vi "Write ACQ Data.vi"(8 "error in (no error)":errorcluster, 10 "ACQ Data":T1, 11 "DriverMasterAsync in":refnum<class "DriverMasterAsync.lvclass">) -> (0 "error out":errorcluster, 3 "DriverMasterAsync out":refnum<class "DriverMasterAsync.lvclass">)   [LabVIEW 2014, in "DriverMasterAsync.lvlib" / "DriverMasterAsync.lvclass"]
uses:
  DriverMasterAsync.lvclass
  APIs/Data Queue/Async Acquisition Data Cluster.ctl
  DriverMasterAsync.lvclass/DriverMasterAsync.ctl
  APIs/Data Queue/WINFAS 2 Data Queue.lvlib
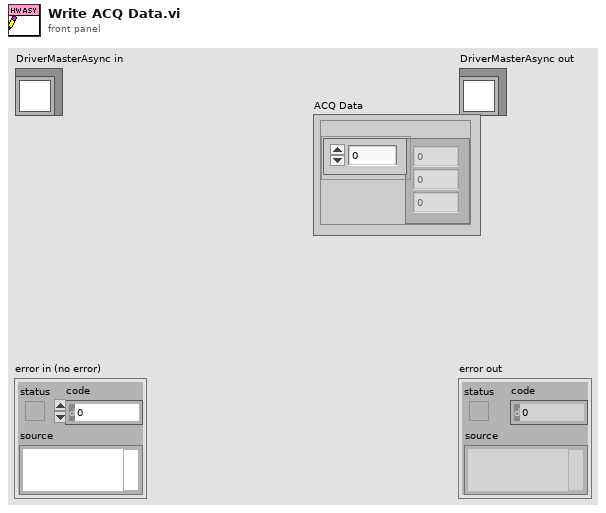
[diagram p1: front panel]
types:
  T1 = typedef "WINFAS 2 Data Queue.lvlib/Async Acquisition Data Cluster.ctl" = cluster{"Data":sgl[]}
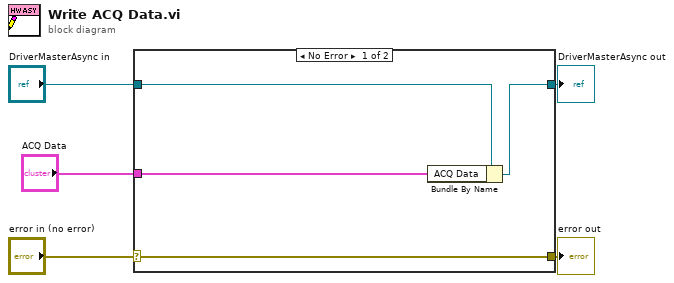
[diagram p0: block diagram]
diagram:
  n1 = case shown="No Error" "error in (no error)" {
    selector: "error in (no error)" -> [w9 w10]
    tunnel: [w9 w10] -> w4
    tunnel: [w7 w11] -> w2
    tunnel: "DriverMasterAsync in" -> [w8 w11]
    tunnel: "ACQ Data" -> [w6 _]
    frame No Error {
      n2 = Bundle By Name(cluster=w8, "ACQ Data"=w6) -> (w7:refnum<class "DriverMasterAsync.lvclass">)
    }
    frame Error {
    }
  }
  "error out" <- w4
  "DriverMasterAsync out" <- w2
